vi "MixingGUIBkup.vi"() -> ()   [LabVIEW 2016]
uses:
  <vilib>/Utility/miscctls.llb/LVStringsAndValuesArrayTypeDef.ctl
  <userlib>/Fluigent/Fluigent MFCS/FluigentMFCS_Full.llb/MFCS_EZ Detect.vi
  <userlib>/Fluigent/Fluigent MFCS/FluigentMFCS_Full.llb/MFCS_EZ Initialization.vi
  Globals/PressuresGlobal.vi
  <userlib>/_OpenG.lib/array/array.llb/Index 1D Array Elements (String)__ogtk.vi
  <vilib>/Utility/file.llb/Write Delimited Spreadsheet (string).vi
  <userlib>/Fluigent/Fluigent MFCS/FluigentMFCS_Full.llb/MFCS_EZ Write Channel Pressure.vi
  <userlib>/_OpenG.lib/array/array.llb/Remove Duplicates from 1D Array (U16)__ogtk.vi
  <userlib>/Fluigent/Fluigent MFCS/FluigentMFCS_Full.llb/MFCS_EZ Close.vi
panel:
  out "Calibration Refs":T1
  in  "Calibration Mode":T2(ring)
  out "Master Pressure Groups":u8[](array[numeric])
  in  "Master Valves":u16(ring) items=["A1", "A2", "A3", "A4", "B1", "B2", "B3", "B4", "B5", "B6", "B7", "B8", "A5"]
  out "Set Pressures":dbl[][](array[numeric])=[[665.1538332158755, 622.4106177021335]]
  out "Ctr Pressure":dbl=199.54651412930238
  in  "stop":bool
  in  "Tab Control":enum32{"Page 1", "Page 2"}(tab)
  in  "Mix Cluster":T3={"Ratio"=[0.6, 0.6, 0.6, 0.6, 0.6, 0.6, 0.6, 0.6], "Mix 2"=[8, 8, 8], "Mix 1"=[0, 0, 0]} {"Mix 1" items=["A1"=0, "A2"=1, "A3"=2, "A4"=3, "A5"=12]; "Mix 2" items=["B5"=8, "B6"=9, "B7"=10, "B8"=11, "A5"=12]}
  out "Ctr Pressure Group":u8=2
  out "Water Mix Pressure Group":u8=1
  in  "Close All Valves":bool
  in  "Odor":u16[](array[ring])=[0, 0, 0, 0, 0, 0, 0, 0] items=["1-pentanol", "3-pentanol", "3-octanol", "2,5-dimethylthiazole", "Add new..."]
  in  "Concentration":u16[](array[ring])=[0, 0, 0, 0, 0, 0, 0, 1] items=["10^-5", "10^-6", "Add new..."]
  in  "Odor Inf Path":path=path "C:/Users/Public/Documents/National Instruments/Fluigent/OdorInf/Data/JB_20171127.txt"
  in  "Append To Odor Inf File":bool=TRUE
  in  "Valves":u16[](array[ring])=[0, 1, 2, 3, 8, 9, 10, 11] items=["A1", "A2", "A3", "A4", "B1", "B2", "B3", "B4", "B5", "B6", "B7", "B8"]
  out "Pressure Group":u8[](array[numeric])=[3, 3, 3, 3, 4, 4, 4, 4]
  in  "Odor Time":dbl[](array[numeric])=[10.0, 10.0, 10.0]
  in  "Water Time":dbl[](array[numeric])=[10.0, 10.0, 10.0]
  in  "Number of Periods":dbl=3.0
  in  "Start Water":dbl=6.0
  out "Experiment Time (Sec)":dbl=46.0
  in  "Calibrate Pressures":bool
  out "Duplicates!":bool
  in  "Zero Pressure":bool
  in  "Water Mix Valve":u16(ring)=12 items=["A1", "A2", "A3", "A4", "B1", "B2", "B3", "B4", "B5", "B6", "B7", "B8", "A5", "A6", "A7", "A8"]
  in  "Ctr Odor Valve":u16(ring)=14 items=["A1", "A2", "A3", "A4", "B1", "B2", "B3", "B4", "B5", "B6", "B7", "B8", "A5", "A6", "A7", "A8"]
  in  "Mix Water Pressure Channel":u16=2
  in  "Control Pressure Channel":u16=1
  out "Current Pressure":dbl[](array[numeric])=[37.23967361450195, 1.893542766571045, 25.247236251831055, 15.779522895812988]
  in  "Manual Default Set Pressures":dbl[](array[numeric])=[199.547, 665.1538332158755, 665.154, 665.154]
  in  "Total Odor Flow":dbl=425.0
  in  "Total Flow Setpoint":dbl=531.25
  out "new file path (Not A Path if cancelled) 2":path
  out "new file path (Not A Path if cancelled)":path
  in  "Master Ratio":dbl[](array[numeric])=[0.6, 0.6]
  in  "Master Mix 2":u16[](array[ring])=[9, 8, 9, 10, 4, 4, 4, 4] items=["B1"=4, "B2"=5, "B3"=6, "B4"=7, "A5"=12]
  in  "Master Mix 1":u16[](array[ring])=[0, 0, 0, 0, 0, 0, 0, 0] items=["A1"=0, "A2"=1, "A3"=2, "A4"=3, "A5"=12]
  in  "Master Water Time":dbl[](array[numeric])=[10.0, 10.0, 10.0, 10.0, 10.0, 10.0, 10.0, 10.0]
  in  "Master Odor Time":dbl[](array[numeric])=[10.0, 10.0, 10.0, 10.0, 10.0, 10.0, 10.0, 10.0]
  out "A5 in Both!":bool
  out "Master Valves":T4=[{"String"="A1", "Value"=0.0}, {"String"="A2", "Value"=1.0}, {"String"="A3", "Value"=2.0}, {"String"="A4", "Value"=3.0}, {"String"="B1", "Value"=4.0}, {"String"="B2", "Value"=5.0}, {"String"="B3", "Value"=6.0}, {"String"="B4", "Value"=7.0}, {"String"="B5", "Value"=8.0}, {"String"="B6", "Value"=9.0}, {"String"="B7", "Value"=10.0}, {"String"="B8", "Value"=11.0}, {"String"="A5", "Value"=12.0}]
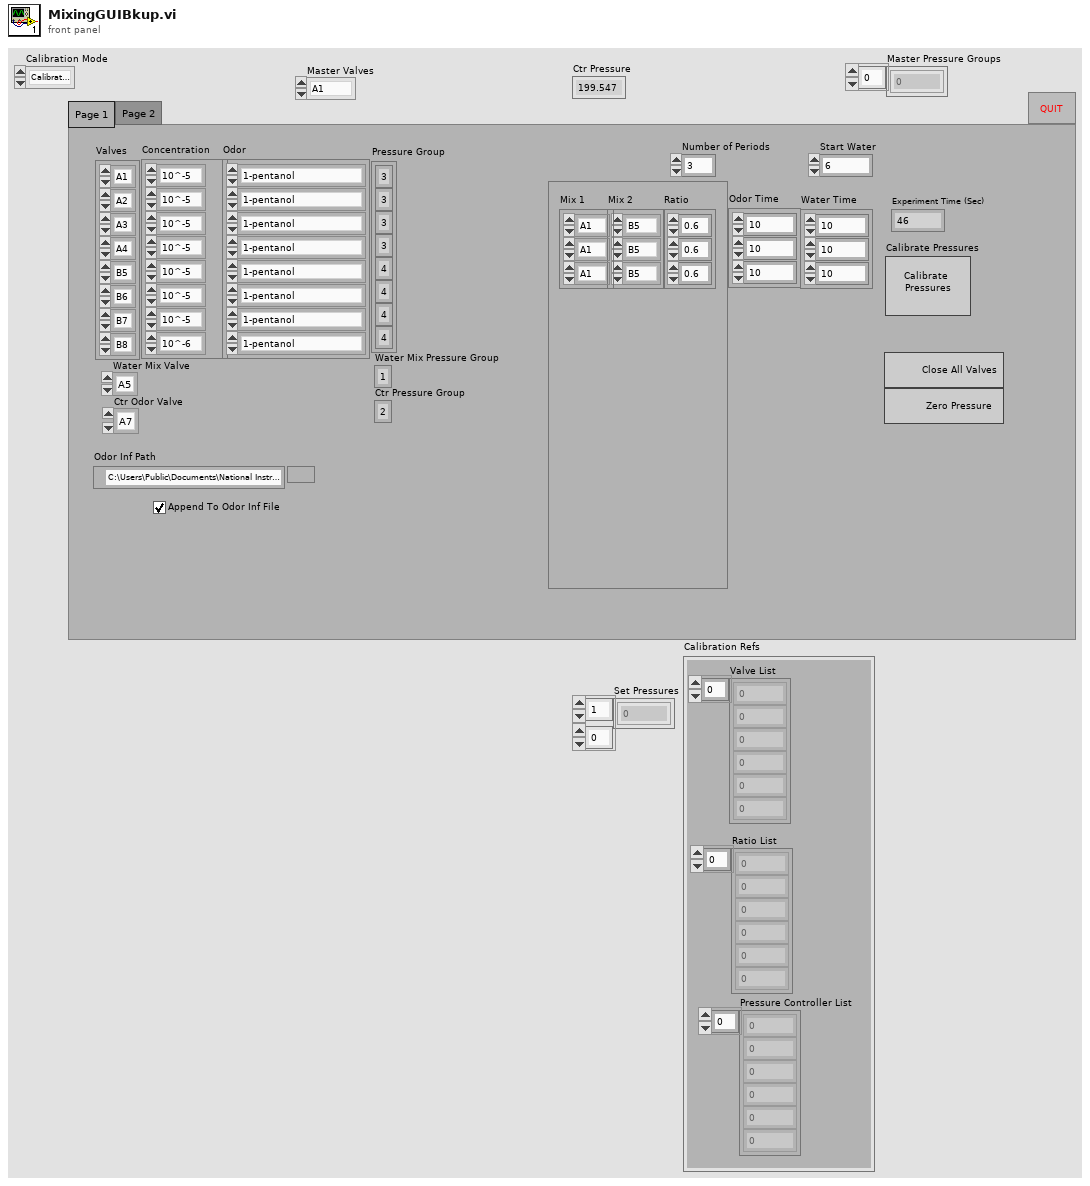
[diagram p1: front panel]
types:
  T1 = cluster{"Pressure Controller List":u8[], "Ratio List":dbl[], "Valve List":u16[]}
  T2 = enum16{"Calibrate All", "Control Only", "Odors Only"}
  T3 = cluster{"Ratio":dbl[], "Mix 2":u16[], "Mix 1":u16[]}
  T4 = typedef "LVStringsAndValuesArrayTypeDef.ctl" = cluster{"String":string, "Value":ext}[]
  T5 = typedef "_EZmfcsSN.ctl" = u16
  T6 = typedef "_EZmfcsRefNum.ctl" = refnum<k1>
  T7 = enum16{"nothing", "All + Keep Old", "All + Remove Old", "Nothing", "New Only", "Nothin3", "Nothing4", "Nothing5", "Cancel"}
  T8 = enum16{"Left Button", "Center Button", "Right Button", "Window Close"}
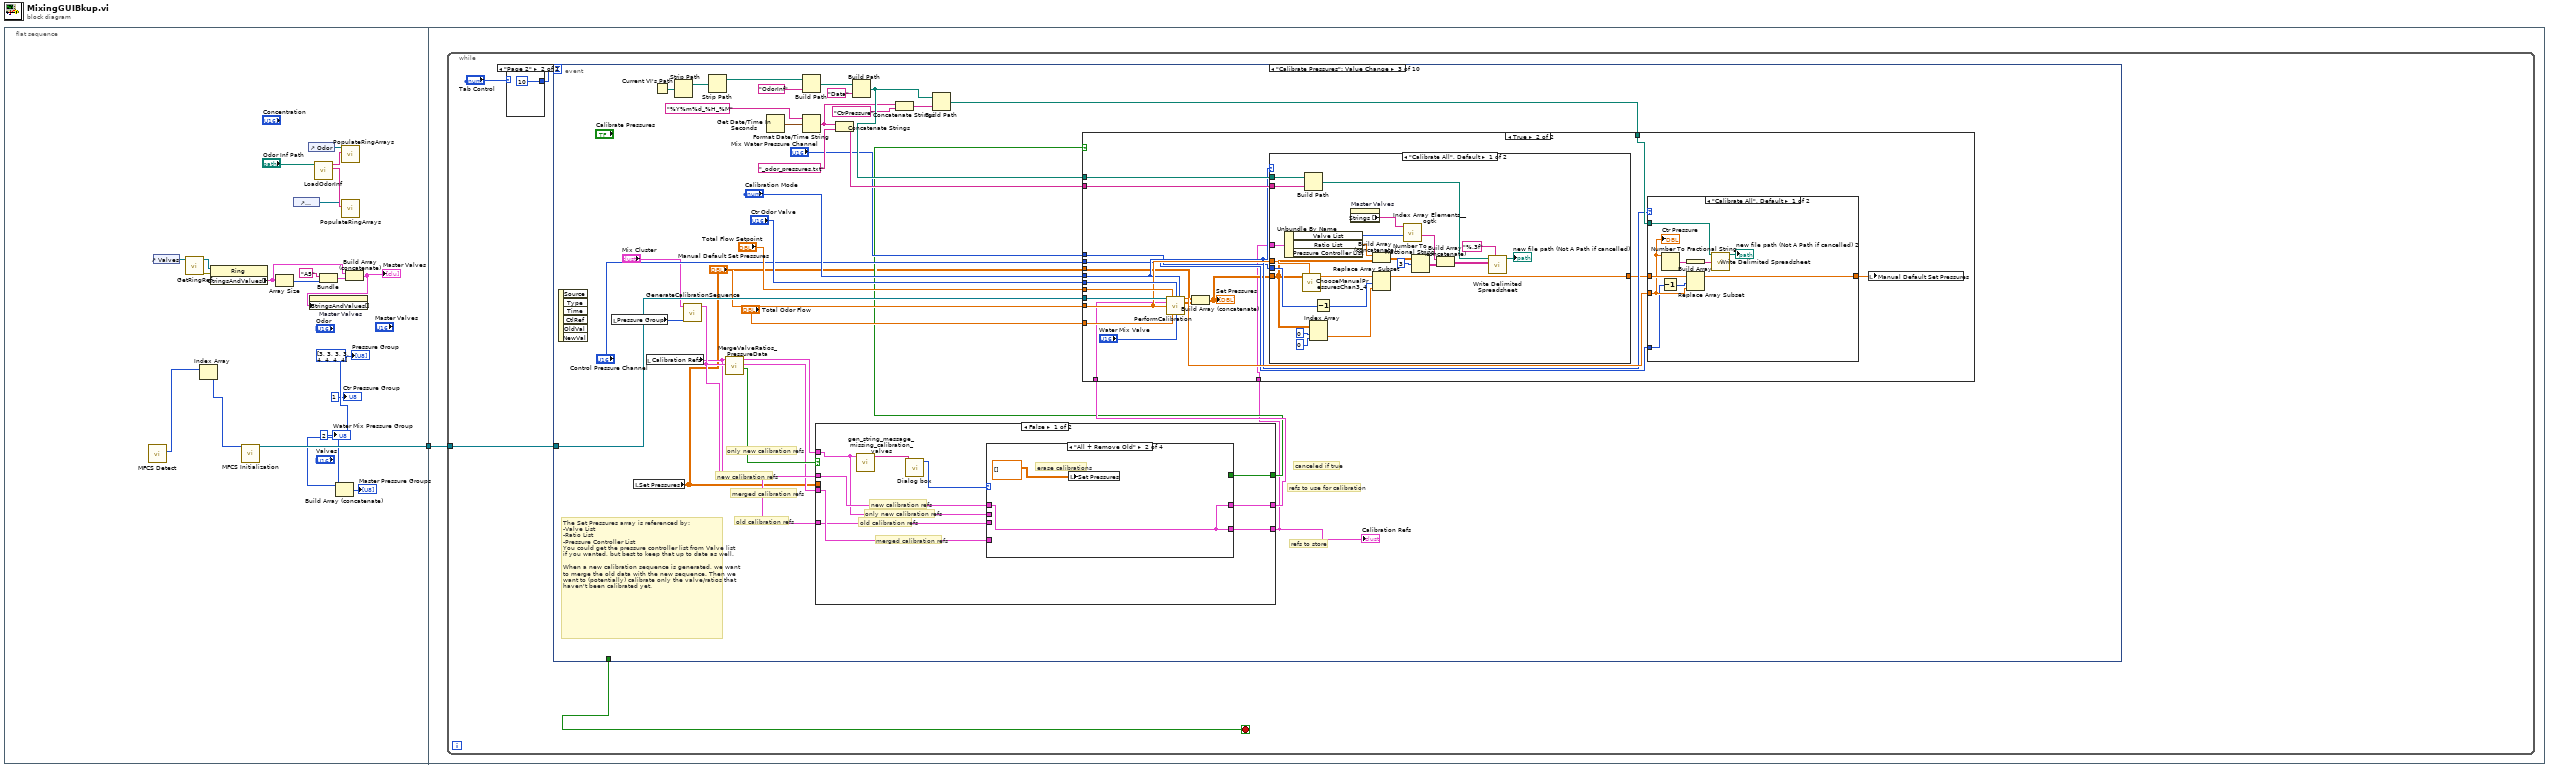
[diagram p0: block diagram]
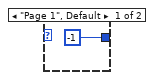
[diagram p2: hidden frame]
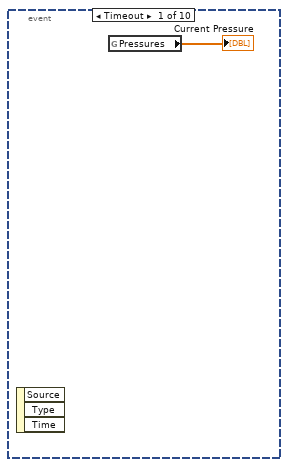
[diagram p3: hidden frame]
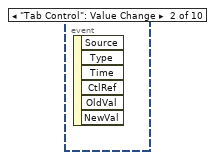
[diagram p4: hidden frame]
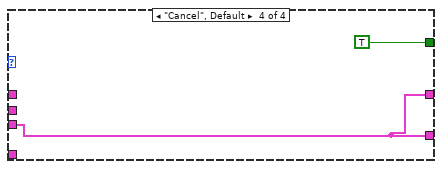
[diagram p10: hidden frame]
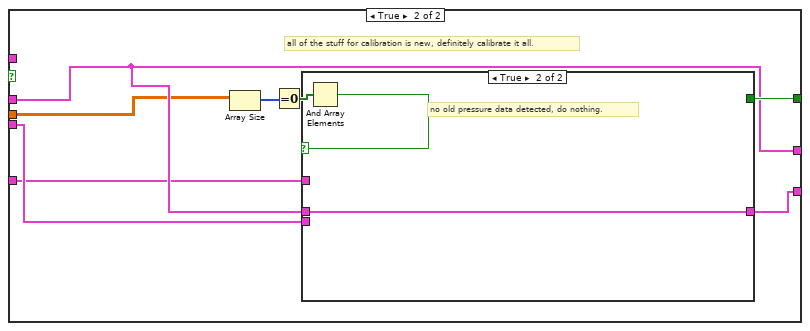
[diagram p11: hidden frame]
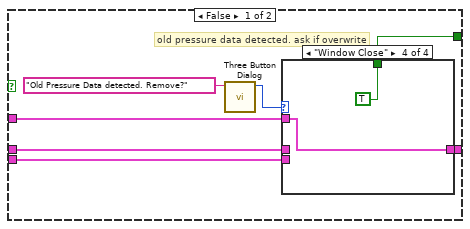
[diagram p12: hidden frame]
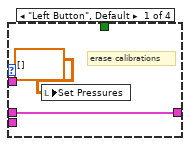
[diagram p13: hidden frame]
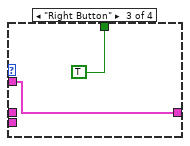
[diagram p15: hidden frame]
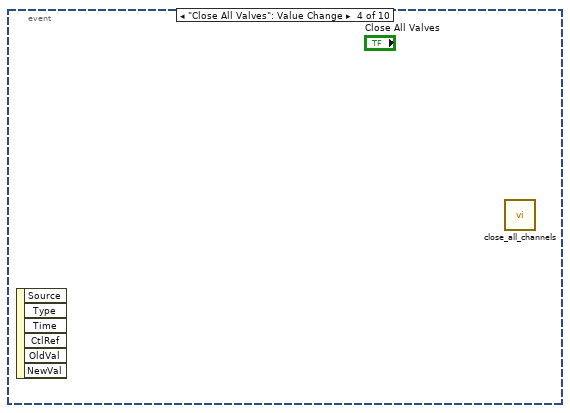
[diagram p16: hidden frame]
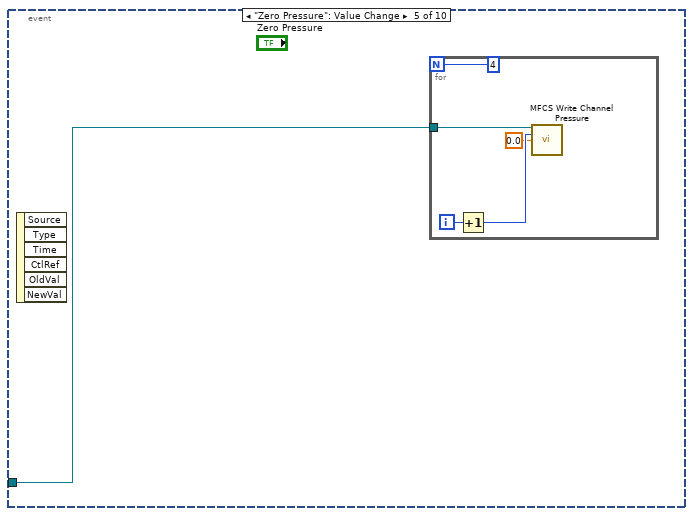
[diagram p17: hidden frame]
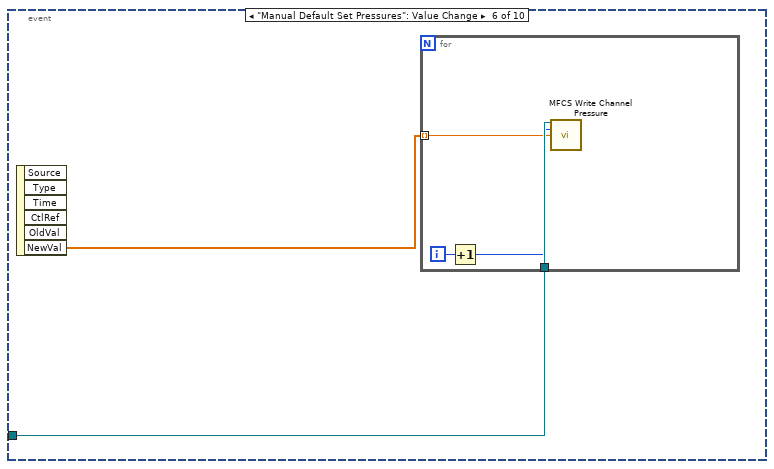
[diagram p18: hidden frame]
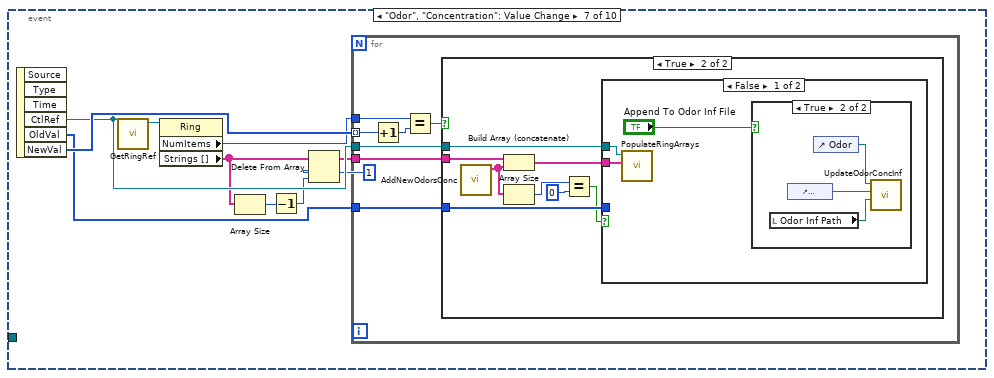
[diagram p19: hidden frame]
diagram:
  n1 = flat-sequence {
    tunnel: [w7] -> w1
    tunnel: w1 -> [w22]
    frame #0 {
      w3 = u8 2 ("Water Mix Pressure Group")
      w5 = u8[] [3, 3, 3, 3, 4, 4, 4, 4] ("Pressure Group")
      n2 = call-poly <userlib>:"MFCS Detect.vi"() -> ("[SN MFCS_EZ]"=w9:T5[])  [unwired: 14 in, 1 out]
      n3 = control-ref of="Valves"() -> (w17:refnum<vi>)
      n4 = call "GetRingRef.vi"("Array Reference"=w17) -> ("error out"=w16:errorcluster, "Ring Reference"=w15:refnum<vi>)  [unwired: 9 in]
      n5 = Index Array(array=w9) -> (element=w8:T5)  [unwired: 1 in]
      n6 = property class="Ring"(reference=w15, error in=w16) -> ("StringsAndValues[]"=w21:T4)  [unwired: 2 out]
      n7 = call-poly <userlib>:"MFCS Initialization.vi"("SN MFCS_EZ"=w8) -> ("MFCS_EZ"=w7:T6)  [unwired: 12 in, 2 out]
      n8 = Array Size(array=w21) -> (size(s)=w19:i32)
      n9 = control-ref of="Concentration"() -> (w13:refnum<vi>)
      n10 = control-ref of="Odor"() -> (w11:refnum<vi>)
      n11 = call "LoadOdorInf.vi"("file path (dialog if empty)"="Odor Inf Path") -> ("Concentration"=w14:string[], "Odor"=w12:string[])  [unwired: 9 in]
      n12 = Bundle("A5", w19) -> (w20:cluster{string, i32})  [unwired: 1 in]
      n13 = Build Array (concatenate)(w5, w3, w3) -> (→"Master Pressure Groups":u8[])
      n14 = call "PopulateRingArrays.vi"("array"=w12, "Array Reference"=w11) -> ()  [unwired: 8 in, 2 out]
      n15 = call "PopulateRingArrays.vi"("array"=w14, "Array Reference"=w13) -> ()  [unwired: 8 in, 2 out]
      n16 = Build Array (concatenate)(w21, w20) -> (w6:T4)
      "Master Valves" <- w6
      n17 = property on="Master Valves" class="Ring (strict)"("StringsAndValues[]"=w6) -> ()  [unwired: 2 in, 2 out]
      "Pressure Group" <- w5
      "Water Mix Pressure Group" <- w3
      "Ctr Pressure Group" <- u8 1 ("Ctr Pressure Group")
    }
    frame #1 {
      n18 = while {
        tunnel: w22 -> [w23]
        stop <- w26 stop-if-true
        n19 = case shown="\"Page 2\"" "Tab Control" {
          tunnel: [-1 10] -> w24
          frame "Page 1", Default {
          }
          frame "Page 2" {
          }
        }
        n20 = event shown="[2] \"Calibrate Pressures\": Value Change" {
          selector: _ -> [_ _ _ _ _ _ _ _ _ _]
          dyn-events: _ -> [_ _ _ _ _ _ _ _ _ _]
          timeout: w24 -> [_ _ _ _ _ _ _ _ _ _]
          tunnel: [_ _ _ _ _ _ _ _ _ TRUE] -> w26
          tunnel: w23 -> [_ _ w48 _ w159 w166 _ _ _ w297]
          event Timeout {
            n21 = event-data() -> ()  [unwired: 1 in, 3 out]
            n22 = global read "PressuresGlobal.vi" "Pressures"() -> (→"Current Pressure":dbl[])
          }
          event "Tab Control": Value Change {
            n23 = event-data() -> ()  [unwired: 1 in, 6 out]
          }
          event "Calibrate Pressures": Value Change {
            # "old calibration refs"
            # "merged calibration refs"
            # "new calibration refs"
            # "only new calibration refs"
            # "canceled if true"
            # "refs to store"
            # "refs to use for calibration"
            # "The Set Pressures array is referenced by:\n-Valve List\n-Ratio List\n-Pressure Controller List\nYou could get the pressure controller list from Valve list if you wanted, but best to keep that up to date as well.\n\nWhen a new calibration sequence is generated, we want to merge the old data with the new sequence. Then we want to (potentially) calibrate only the valve/ratios that haven't been calibrated yet."
            n24 = event-data() -> ()  [unwired: 1 in, 6 out]
            n25 = local read "Pressure Group"() -> (w46:u8[])
            n26 = local read "Set Pressures"() -> (w31:dbl[][])
            n27 = local read "Calibration Refs"() -> (w32:T1)
            n28 = Current VI's Path() -> (path=w57:path)
            n29 = Strip Path(path=w57) -> (stripped path=w45:path)  [unwired: 1 out]
            n30 = call "GenerateCalibrationSequence.vi"("Pressure Group"=w46, "Mix Cluster"="Mix Cluster") -> ("Calibration Refs"=w36:T1)  [unwired: 9 in]
            n31 = Strip Path(path=w45) -> (stripped path=w44:path)  [unwired: 1 out]
            n32 = call "MergeValveRatios_PressureData.vi"("New Calibration Refs"=w36, "Old Calibration Refs"=w32) -> ("None already calibrated?"=w38:bool, "Merged Calibration Refs"=w35:T1, "Only New Calibration Refs"=w37:T1)  [unwired: 7 in]
            n33 = Get Date/Time In Seconds() -> (seconds since 1Jan1904=w60:timestamp)
            n34 = Build Path(base path=w44, name or relative path="OdorInf") -> (appended path=w56:path)
            n35 = Format Date/Time String(time format string (%c)="%Y%m%d_%H_%M", seconds (now)=w60) -> (date/time string=w52:string)  [unwired: 1 in]
            n36 = case shown="False" w38 {
              tunnel: w37 -> [w123 _]
              tunnel: w36 -> [w124 w139]
              tunnel: w35 -> [w122 w137]
              tunnel: [w121 w138] -> w30
              tunnel: [w120 w139] -> w34
              tunnel: [w119 w140] -> w33
              tunnel: w32 -> [w118 w136]
              tunnel: w31 -> [_ w135]
              frame False {
                # "old calibration refs"
                # "merged calibration refs"
                # "new calibration refs"
                # "only new calibration refs"
                n37 = call "gen_string_message_missing_calibration_valves.vi"("Missing Calibration Refs"=w123) -> ("String"=w126:string)  [unwired: 9 in]
                n38 = call "Dialog box.vi"("Missing Str"=w126) -> ("Response"=w125:T7)  [unwired: 9 in]
                n39 = case shown="\"All + Remove Old\"" w125 {
                  tunnel: w124 -> [w127 w129 _ _]
                  tunnel: w123 -> [_ _ w132 _]
                  tunnel: w122 -> [w128 _ w131 _]
                  tunnel: [w128 w129 w131 w133] -> w121
                  tunnel: [w127 w129 w132 w133] -> w120
                  tunnel: [_ _ _ TRUE] -> w119
                  tunnel: w118 -> [_ _ _ w133]
                  frame "All + Keep Old" {
                  }
                  frame "All + Remove Old" {
                    # "erase calibrations"
                    n40 = local write "Set Pressures"(dbl[][] []) -> ()
                  }
                  frame "New Only" {
                  }
                  frame "Cancel", Default {
                  }
                }
              }
              frame True {
                # "all of the stuff for calibration is new, definitely calibrate it all."
                n41 = Array Size(array=w135) -> (size(s)=w143:i32[])
                n42 = Equal To 0?(x=w143) -> (x = 0?=w142:bool[])
                n43 = And Array Elements(Boolean array=w142) -> (logical AND=w141:bool)
                n44 = case shown="True" w141 {
                  tunnel: [w148 _] -> w140
                  tunnel: w139 -> [w147 w158]
                  tunnel: [w146 w158] -> w138
                  tunnel: w137 -> [w145 _]
                  tunnel: w136 -> [w144 _]
                  frame False {
                    # "old pressure data detected. ask if overwrite"
                    n45 = call <vilib>:"Three Button Dialog.vi"("message"="Old Pressure Data detected. Remove?") -> ("Which Button?"=w149:T8)  [unwired: 10 in]
                    n46 = case shown="\"Window Close\"" w149 {
                      tunnel: [_ _ TRUE TRUE] -> w148
                      tunnel: w147 -> [w151 _ _ _]
                      tunnel: [w151 w153 w154 w156] -> w146
                      tunnel: w145 -> [_ w153 _ _]
                      tunnel: w144 -> [_ _ w154 w156]
                      frame "Left Button", Default {
                        # "erase calibrations"
                        n47 = local write "Set Pressures"(dbl[][] []) -> ()
                      }
                      frame "Center Button" {
                        # "don't overwrite"
                      }
                      frame "Right Button" {
                      }
                      frame "Window Close" {
                      }
                    }
                  }
                  frame True {
                    # "no old pressure data detected, do nothing."
                  }
                }
              }
            }
            "Calibration Refs" <- w30
            n48 = Concatenate Strings(w52, "_odor_pressures.txt" ("string")) -> (w54:string)
            n49 = Build Path(base path=w56, name or relative path="Data") -> (appended path=w53:path)
            n50 = Concatenate Strings(w52, "CtrPressure" ("string")) -> (w50:string)
            n51 = Build Path(base path=w53, name or relative path=w50) -> (appended path=w49:path)
            n52 = case shown="True" w33 {
              tunnel: "Total Odor Flow" -> [_ w83]
              tunnel: "Total Flow Setpoint" -> [_ w82]
              tunnel: w54 -> [_ w81]
              tunnel: w53 -> [_ w80]
              tunnel: w49 -> [_ w79]
              tunnel: w48 -> [_ w78]
              tunnel: "Ctr Odor Valve" -> [_ w77]
              tunnel: "Manual Default Set Pressures" -> [_ w74]
              tunnel: "Calibration Mode" -> [_ w73]
              tunnel: "Control Pressure Channel" -> [_ w71]
              tunnel: "Mix Water Pressure Channel" -> [_ w69]
              tunnel: w34 -> [_ w68]
              tunnel: w31 -> [_ w66]
              tunnel: w30 -> [_ w64]
              frame False {
              }
              frame True {
                n53 = call "PerformCalibration.vi"("MFCS_EZ"=w78, "Total Flow Setpoint"=w82, "Ctr Water Valve"=w77, "Calibration Mode"=w73, "Calibration Refs"=w68, "Manual Default Set Pressures"=w74, "Total Odor Flow"=w83, "Water Mix Valve"="Water Mix Valve") -> ("Ctr Pressure"=w75:dbl, "Set Pressures"=w67:dbl[][])  [unwired: 6 in]
                n54 = Build Array (concatenate)(w66, w67) -> (w65:dbl[][])
                "Set Pressures" <- w65
                n55 = case shown="\"Calibrate All\", Default" w73 {
                  tunnel: w81 -> [w103 _]
                  tunnel: w80 -> [w101 _]
                  tunnel: w65 -> [w89 _]
                  tunnel: w74 -> [w100 w107]
                  tunnel: [w93 w107] -> w72
                  tunnel: w69 -> [w96 _]
                  tunnel: w64 -> [w92 _]
                  frame "Calibrate All", Default {
                    n56 = Unbundle By Name(w92) -> ("Valve List"=w91:u16[], "Ratio List"=w88:dbl[])  [unwired: 1 out]
                    n57 = call "ChooseManualPressuresChan3_4.vi"("Manual Pressure In"=w100, "Set Pressures"=w89) -> ("Manual Pressure"=w97:dbl[])  [unwired: 9 in]
                    n58 = Build Path(base path=w101, name or relative path=w103) -> (appended path=w102:path)
                    n59 = Index Array(array=w89, index (row)=0, index (col)=0 ("disabled index (col)")) -> (element=w94:dbl)
                    n60 = Decrement(x=w96) -> (x-1=w95:u16)
                    n61 = property on="Master Valves" class="Ring (strict)"() -> ("Strings []"=w90:string[])  [unwired: 2 in, 2 out]
                    n62 = Build Array (concatenate)(w88, w89) -> (w87:dbl[][])
                    n63 = Replace Array Subset(array=w97, new element=w94, index=w95) -> (w93:dbl[])
                    n64 = call-poly <userlib>:"Index Array Elements__ogtk.vi"("indices"=w91, "array"=w90) -> ("elements"=w85:string[])  [unwired: 9 in]
                    n65 = Number To Fractional String(number=w87, width (-)=i16 3) -> (F-format string=w86:string[][])  [unwired: 2 in]
                    n66 = Build Array (concatenate)(w85, w86) -> (w84:string[][])
                    n67 = call-poly <vilib>:"Write Delimited Spreadsheet.vi"("file path (dialog if empty)"=w102, "format (%s)"="%.3f" ("format (%.3f)"), "2D data"=w84) -> ("new file path (Not A Path if cancelled)"=→"new file path (Not A Path if cancelled)":path)  [unwired: 11 in, 1 out]
                  }
                  frame "Control Only" {
                  }
                }
                n68 = case shown="\"Calibrate All\", Default" w73 {
                  tunnel: w79 -> [w116 _]
                  tunnel: w75 -> [w111 _]
                  tunnel: w72 -> [w112 w117]
                  tunnel: w71 -> [w110 _]
                  tunnel: [w108 w117] -> w70
                  frame "Calibrate All", Default {
                    n69 = Decrement(x=w110) -> (x-1=w109:u16)
                    n70 = Number To Fractional String(number=w111) -> (F-format string=w115:string)  [unwired: 3 in]
                    n71 = Build Array(w115) -> (w114:string[])
                    n72 = Replace Array Subset(array=w112, new element=w111, index=w109) -> (w108:dbl[])
                    n73 = call-poly <vilib>:"Write Delimited Spreadsheet.vi"("file path (dialog if empty)"=w116, "1D data"=w114) -> ("new file path (Not A Path if cancelled)"=→"new file path (Not A Path if cancelled) 2":path)  [unwired: 12 in, 1 out]
                    "Ctr Pressure" <- w111
                  }
                  frame "Odors Only" {
                  }
                }
                n74 = local write "Manual Default Set Pressures"(w70) -> ()
              }
            }
          }
          event "Close All Valves": Value Change {
            n75 = event-data() -> ()  [unwired: 1 in, 6 out]
            n76 = call "close_all_channels.vi"() -> ()  [unwired: 12 in]
          }
          event "Zero Pressure": Value Change {
            n77 = event-data() -> ()  [unwired: 1 in, 6 out]
            n78 = for {
              N: 4 -> [_]
              tunnel: w159 -> [w161]
              i -> [w164]
              n79 = Increment(x=w164) -> (x+1=w163:i32)
              n80 = call-poly <userlib>:"MFCS Write Channel Pressure.vi"("MFCS_EZ"=w161, "Channel Number (default=1)"=w163, "Pressure (mBar)"=0.0) -> ()  [unwired: 11 in, 2 out]
            }
          }
          event "Manual Default Set Pressures": Value Change {
            n81 = event-data() -> ("NewVal"=w165:dbl[])  [unwired: 1 in, 5 out]
            n82 = for {
              tunnel: w166 -> [w170]
              tunnel: w165 -> [w169] mode=indexing
              i -> [w168]
              n83 = Increment(x=w168) -> (x+1=w167:i32)
              n84 = call-poly <userlib>:"MFCS Write Channel Pressure.vi"("MFCS_EZ"=w170, "Channel Number (default=1)"=w167, "Pressure (mBar)"=w169) -> ()  [unwired: 11 in, 2 out]
            }
          }
          event "Odor", "Concentration": Value Change {
            n85 = event-data() -> ("CtlRef"=w177:refnum<vi>, "OldVal"=w171:u16[], "NewVal"=w179:u16[])  [unwired: 1 in, 3 out]
            n86 = call "GetRingRef.vi"("Array Reference"=w177) -> ("Ring Reference"=w180:refnum<vi>)  [unwired: 9 in, 1 out]
            n87 = property class="Ring"(reference=w180) -> ("NumItems"=w178:u32, "Strings []"=w176:string[])  [unwired: 1 in, 2 out]
            n88 = Array Size(array=w176) -> (size(s)=w175:i32)
            n89 = Decrement(x=w175) -> (x-1=w172:i32)
            n90 = Delete From Array(array=w176, length=1, index=w172) -> (array with subset deleted=w173:string[])  [unwired: 1 out]
            n91 = for {
              tunnel: w179 -> [w187] mode=indexing
              tunnel: w178 -> [w186]
              tunnel: w177 -> [w184]
              tunnel: w173 -> [w183]
              tunnel: w171 -> [w181]
              n92 = Increment(x=w187) -> (x+1=w182:u16)
              n93 = Equal?(x=w186, y=w182) -> (x = y?=w185:bool)
              n94 = case shown="True" w185 {
                tunnel: w184 -> [_ w194]
                tunnel: w183 -> [_ w195]
                tunnel: w181 -> [_ w193]
                frame False {
                }
                frame True {
                  n95 = call "AddNewOdorsConc.vi"() -> ("To Add Out"=w191:string[])  [unwired: 10 in]
                  n96 = Build Array (concatenate)(w195, w191) -> (w192:string[])
                  n97 = Array Size(array=w191) -> (size(s)=w190:i32)
                  n98 = Equal?(x=w190, y=0 ("size(s)")) -> (x = y?=w188:bool)
                  n99 = case shown="False" w188 {
                    tunnel: w194 -> [w198 w203]
                    tunnel: w193 -> [_ w202]
                    tunnel: w192 -> [w197 _]
                    frame False {
                      n100 = call "PopulateRingArrays.vi"("array"=w197, "Array Reference"=w198) -> ()  [unwired: 8 in, 2 out]
                      n101 = case shown="True" "Append To Odor Inf File" {
                        frame False {
                        }
                        frame True {
                          n102 = local read "Odor Inf Path"() -> (w199:path)
                          n103 = control-ref of="Concentration"() -> (w201:refnum<vi>)
                          n104 = control-ref of="Odor"() -> (w200:refnum<vi>)
                          n105 = call "UpdateOdorConcInf.vi"("Path"=w199, "Concentration Ref"=w201, "Odor Ref"=w200) -> ()  [unwired: 9 in]
                        }
                      }
                    }
                    frame True {
                      n106 = property class="Arr (strict)"(reference=w203, "Value"=w202) -> ()  [unwired: 1 in, 2 out]
                    }
                  }
                }
              }
            }
          }
          event "Valves": Value Change {
            # "greater than 0 means there are duplicates"
            n107 = event-data() -> ("NewVal"=w204:u16[])  [unwired: 1 in, 5 out]
            n108 = call-poly <userlib>:"Remove Duplicates from 1D Array__ogtk.vi"("Input Array"=w204) -> ("indices of removed elements"=w208:i32[])  [unwired: 1 out]
            n109 = Array Size(array=w208) -> (size(s)=w206:i32)
            n110 = Greater?(x=w206, y=0 ("x")) -> (0:w205:bool)
            "Duplicates!" <- w205
            n111 = property on="Duplicates!" class="Bool (strict)"("Blinking"=w205, "Visible"=w205) -> ()  [unwired: 2 in, 2 out]
            n112 = case shown="False" w205 {
              tunnel: w204 -> [w222 _]
              frame False {
                w236 = 4 ("index")
                n113 = control-ref of="Valves"() -> (w239:refnum<vi>)
                n114 = call "GetRingRef.vi"("Array Reference"=w239) -> ("error out"=w237:errorcluster, "Ring Reference"=w238:refnum<vi>)  [unwired: 9 in]
                n115 = local read "Mix Cluster"() -> (w210:T3)
                n116 = property class="Ring"(reference=w238, error in=w237) -> ("StringsAndValues[]"=w212:T4)  [unwired: 2 out]
                n117 = Unbundle By Name(w210) -> ("Mix 1"=w209:u16[])
                n118 = for {
                  tunnel: w222 -> [w241] mode=indexing
                  tunnel: w212 -> [w242]
                  tunnel: [w240] -> w225 mode=indexing
                  n119 = Index Array(array=w242, index=w241) -> (element=w240:cluster{"String":string, "Value":ext})
                }
                n120 = Array Size(array=w212) -> (size(s)=w211:i32)
                n121 = Split 1D Array(array=w222, index=w236) -> (first subarray=w218:u16[], second subarray=w219:u16[])
                n122 = Array Size(array=w209) -> (size(s)=w215:i32)
                n123 = Index Array(array=w218, index=0) -> (element=w217:u16)
                n124 = Index Array(array=w219, index=0) -> (element=w216:u16)
                n125 = Bundle("A5", w211) -> (w234:cluster{string, i32})  [unwired: 1 in]
                n126 = control-ref of="Mix 1"() -> (w223:refnum<vi>)
                n127 = control-ref of="Mix 2"() -> (w224:refnum<vi>)
                n128 = Initialize Array(w217, w215) -> (w214:u16[])
                n129 = Initialize Array(w216, w215) -> (w213:u16[])
                n130 = Split 1D Array(array=w225, index=w236) -> (first subarray=w232:cluster{"String":string, "Value":ext}[], second subarray=w233:cluster{"String":string, "Value":ext}[])
                n131 = property class="Arr (strict)"(reference=w223, "Value"=w214) -> ()  [unwired: 1 in, 2 out]
                n132 = property class="Arr (strict)"(reference=w224, "Value"=w213) -> ()  [unwired: 1 in, 2 out]
                n133 = Build Array (concatenate)(w232, w234) -> (w226:cluster{"String":string, "Value":ext}[])
                n134 = Build Array (concatenate)(w233, w234) -> (w227:cluster{"String":string, "Value":ext}[])
                n135 = call "GetRingRef.vi"("Array Reference"=w223) -> ("error out"=w230:errorcluster, "Ring Reference"=w231:refnum<vi>)  [unwired: 9 in]
                n136 = call "GetRingRef.vi"("Array Reference"=w224) -> ("error out"=w228:errorcluster, "Ring Reference"=w229:refnum<vi>)  [unwired: 9 in]
                n137 = property class="Ring"(reference=w231, error in=w230, "StringsAndValues[]"=w226) -> ()  [unwired: 2 out]
                n138 = property class="Ring"(reference=w229, error in=w228, "StringsAndValues[]"=w227) -> ()  [unwired: 2 out]
              }
              frame True {
              }
            }
          }
          event "Number of Periods", "Mix Cluster.Mix 1", "Mix Cluster.Mix 2": Value Change {
            n139 = event-data() -> ()  [unwired: 1 in, 6 out]
            n140 = local read "Mix Cluster"() -> (w251:T3)
            n141 = Unbundle By Name(w251) -> ("Mix 2"=w244:u16[], "Mix 1"=w243:u16[])  [unwired: 1 out]
            n142 = local read "Master Valves"() -> (w280:T4)
            n143 = control-ref of="Water Time"() -> (w288:refnum<vi>)
            n144 = control-ref of="Odor Time"() -> (w296:refnum<vi>)
            n145 = control-ref of="Ratio"() -> (w268:refnum<vi>)
            n146 = control-ref of="Mix 1"() -> (w281:refnum<vi>)
            n147 = control-ref of="Mix 2"() -> (w282:refnum<vi>)
            n148 = Array Size(array=w280) -> (size(s)=w270:i32)
            n149 = Add Array Elements(numeric array="Water Time") -> (sum=w261:dbl)
            n150 = Add Array Elements(numeric array="Odor Time") -> (sum=w260:dbl)
            n151 = call "MakeArrayRightSize.vi"("Size"="Number of Periods", "Master Array In"="Master Water Time", "Array"="Water Time", "reference"=w288) -> ("Array Out"=w289:variant[], "Master Array Out"=w290:variant[])  [unwired: 6 in]
            n152 = call "MakeArrayRightSize.vi"("Size"="Number of Periods", "Master Array In"="Master Odor Time", "Array"="Odor Time", "reference"=w296) -> ("Array Out"=w294:variant[], "Master Array Out"=w292:variant[])  [unwired: 6 in]
            n153 = call "MakeArrayRightSize.vi"("Size"="Number of Periods", "Master Array In"="Master Ratio", "reference"=w268) -> ("Array Out"=w266:variant[], "Master Array Out"=w267:variant[])  [unwired: 7 in]
            n154 = call "MakeArrayRightSize.vi"("Size"="Number of Periods", "Master Array In"="Master Mix 1", "Array"=w243, "reference"=w281) -> ("Array Out"=w250:variant[], "Master Array Out"=w249:variant[])  [unwired: 6 in]
            n155 = call "MakeArrayRightSize.vi"("Size"="Number of Periods", "Master Array In"="Master Mix 2", "Array"=w244, "reference"=w282) -> ("Array Out"=w254:variant[], "Master Array Out"=w253:variant[])  [unwired: 6 in]
            n156 = Variant To Data(type="Water Time", Variant=w290) -> (data=w285:dbl[])  [unwired: 1 in, 1 out]
            n157 = Variant To Data(type="Water Time", Variant=w289) -> (data=w286:dbl[])  [unwired: 1 in, 1 out]
            n158 = Variant To Data(type="Odor Time", Variant=w292) -> (data=w291:dbl[])  [unwired: 1 in, 1 out]
            n159 = Variant To Data(type="Odor Time", Variant=w294) -> (data=w293:dbl[])  [unwired: 1 in, 1 out]
            n160 = Variant To Data(Variant=w249) -> (data=w248:u16[])  [unwired: 2 in, 1 out]
            n161 = Variant To Data(type=w243, Variant=w250) -> (data=w247:u16[])  [unwired: 1 in, 1 out]
            n162 = Variant To Data(Variant=w253) -> (data=w252:u16[])  [unwired: 2 in, 1 out]
            n163 = Variant To Data(type=w244, Variant=w254) -> (data=w255:u16[])  [unwired: 1 in, 1 out]
            n164 = Add(x=w261, y=w260) -> (x+y=w259:dbl)
            n165 = Variant To Data(type="Master Ratio", Variant=w267) -> (data=w246:dbl[])  [unwired: 1 in, 1 out]
            n166 = Variant To Data(Variant=w266) -> (data=w265:dbl[])  [unwired: 2 in, 1 out]
            n167 = Decrement(x=w270) -> (x-1=w269:i32)
            n168 = local write "Master Water Time"(w285) -> ()
            n169 = local write "Water Time"(w286) -> ()
            n170 = local write "Master Odor Time"(w291) -> ()
            n171 = local write "Odor Time"(w293) -> ()
            n172 = local write "Master Ratio"(w265) -> ()
            n173 = local write "Master Mix 1"(w248) -> ()
            n174 = local write "Master Mix 2"(w252) -> ()
            n175 = Search 1D Array(1D array=w244, element=w269) -> (index of element=w279:i32)  [unwired: 1 in]
            n176 = Search 1D Array(1D array=w243, element=w269) -> (index of element=w276:i32)  [unwired: 1 in]
            n177 = Add(x="Start Water", y=w259) -> (x+y=→"Experiment Time (Sec)":dbl)
            n178 = Equal?(x=w279, y=-1) -> (x = y?=w275:bool)
            n179 = Equal?(x=w276, y=-1) -> (x = y?=w274:bool)
            n180 = Bundle By Name(cluster=w251, "Ratio"=w246, "Mix 2"=w255, "Mix 1"=w247) -> (w256:T3)
            n181 = local write "Mix Cluster"(w256) -> ()
            n182 = Not(x=w275) -> (.not. x?=w271:bool)
            n183 = Not(x=w274) -> (.not. x?=w272:bool)
            n184 = And(x=w271, y=w272) -> (x .and. y?=w273:bool)
            "A5 in Both!" <- w273
            n185 = property on="A5 in Both!" class="Bool (strict)"("Visible"=w273, "Blinking"=w273) -> ()  [unwired: 2 in, 2 out]
          }
          event "stop": Value Change {
            n186 = event-data() -> ()  [unwired: 1 in, 6 out]
            n187 = call-poly <userlib>:"MFCS Close.vi"("MFCS_EZ"=w297) -> ()  [unwired: 14 in, 1 out]
          }
        }
      }
    }
  }
